vi "CRYUnflatten Curve Test Info.vi"(11 "Falattend test info":string) -> (0 "Error?":bool=TRUE, 2 "unflattened test info data":cluster{"Original Res":string, "Steps":i32})   [LabVIEW 2013]
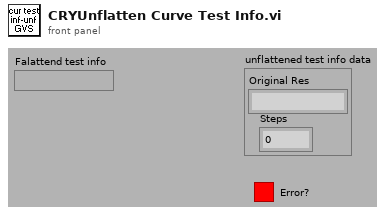
[diagram p1: front panel]
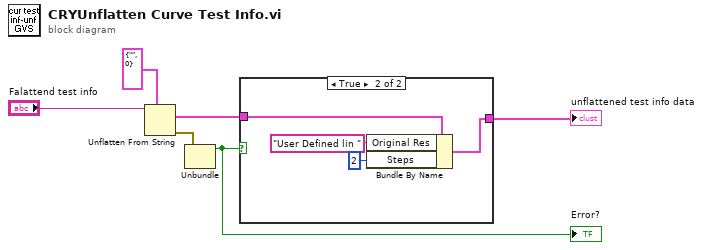
[diagram p0: block diagram]
diagram:
  n1 = Unflatten From String(type=cluster{"Original Res":string, "Steps":i32} {"Original Res"="", "Steps"=0} ("Cal Test Info"), binary string="Falattend test info") -> (value=w3:cluster{"Original Res":string, "Steps":i32}, error out=w5:errorcluster)  [unwired: 1 in, 3 out]
  n2 = Unbundle(w5) -> ("status"=w4:bool)  [unwired: 2 out]
  "Error?" <- w4
  n3 = case shown="True" w4 {
    tunnel: w3 -> [w7 w11]
    tunnel: [w7 w10] -> w1
    frame False {
    }
    frame True {
      n4 = Bundle By Name(cluster=w11, "Original Res"="User Defined lin ", "Steps"=2) -> (w10:cluster{"Original Res":string, "Steps":i32})
    }
  }
  "unflattened test info data" <- w1
